vi "ReadB.vi"() -> ()   [LabVIEW 2015]
uses:
  ESLSCDLL.dll
panel:
  out "Data":u8=255
  in  "Offset":u32
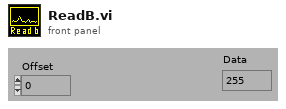
[diagram p1: front panel]
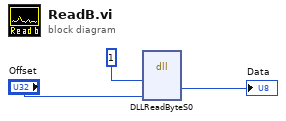
[diagram p0: block diagram]
diagram:
  n1 = dll-call lib="C:/ENTW/PCIE/64bit/lv64/1cam/board.vis/ESLSCDLL.dll" fn="DLLReadByteS0"("drv"=u32 1, "PortOff"="Offset") -> ("data"=→"Data":u8)  [unwired: 7 in, 2 out]
